vi "Get 430 Rate.vi"(5 "Field [T]":dbl, 7 "Override field?":bool, 8 "error in (no error)":errorcluster, 11 "VISA session":refnum<visa-resource-name>="GPIB0::22::INSTR") -> (0 "error out":errorcluster, 2 "Slew Rate [T/min]":dbl, 3 "VISA session out":refnum<visa-resource-name>="GPIB0::22::INSTR")   [LabVIEW 2021]
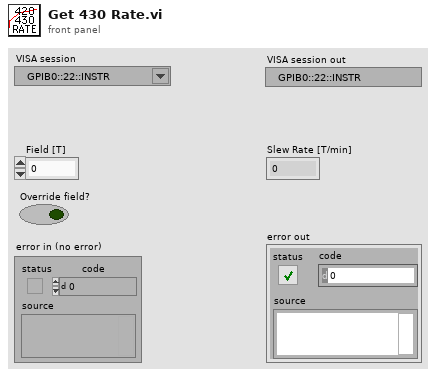
[diagram p1: front panel]
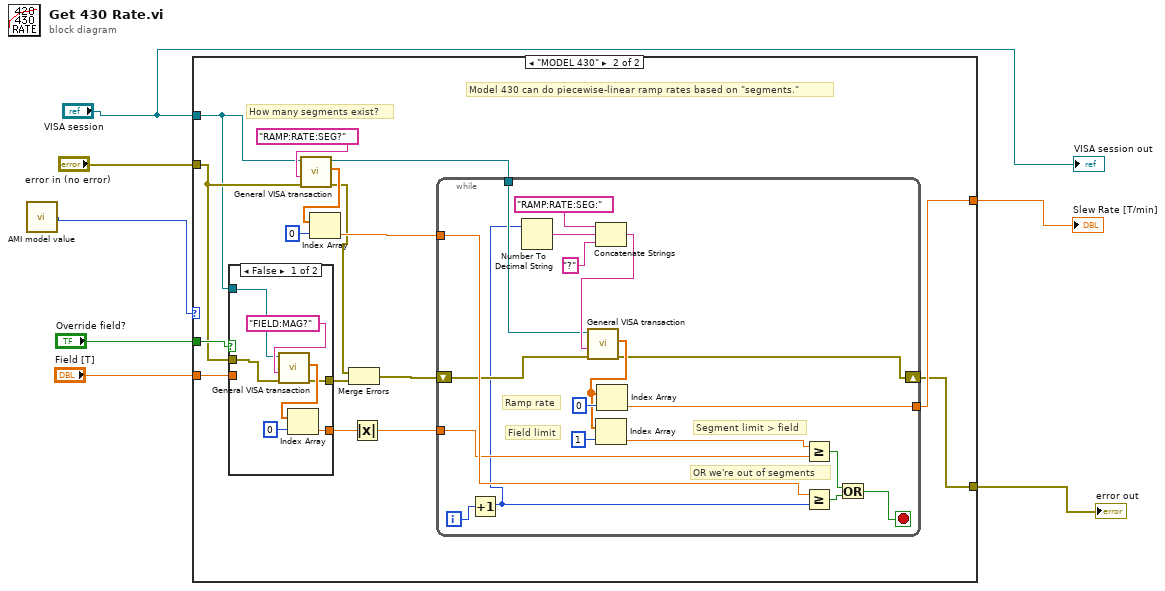
[diagram p0: block diagram]
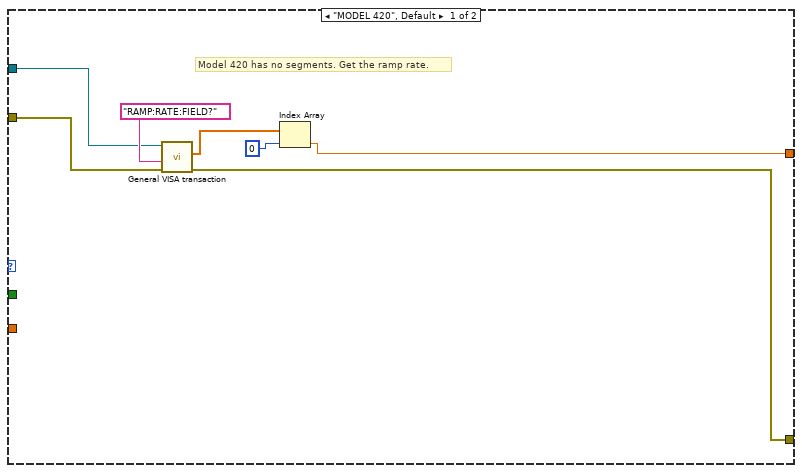
[diagram p2: hidden frame]
diagram:
  n1 = call "AMI model value.vi"() -> ("AMI Model 2"=w1:enum16{"MODEL 420", "MODEL 430"})  [unwired: 2 in]
  n2 = case shown="\"MODEL 430\"" w1 {
    tunnel: "VISA session" -> [w13 w20]
    tunnel: "error in (no error)" -> [w12 w25]
    tunnel: "Field [T]" -> [_ w29]
    tunnel: [w11 w15] -> w5
    tunnel: [w8 w16] -> w3
    tunnel: "Override field?" -> [_ w30]
    frame "MODEL 420", Default {
      # "Model 420 has no segments. Get the ramp rate."
      n3 = call "General VISA transaction.vi"("error in (no error)"=w12, "Command String"="RAMP:RATE:FIELD?", "VISA Session"=w13) -> ("error out"=w11:errorcluster, "Measurement"=w9:dbl[])  [unwired: 3 in, 4 out]
      n4 = Index Array(array=w9, index=0) -> (element=w8:dbl)
    }
    frame "MODEL 430" {
      # "How many segments exist?"
      # "Model 430 can do piecewise-linear ramp rates based on \"segments.\""
      n5 = case shown="False" w30 {
        tunnel: w29 -> [_ w58]
        tunnel: w25 -> [w55 w57]
        tunnel: [w52 w58] -> w18
        tunnel: [w51 w57] -> w23
        tunnel: w20 -> [w50 _]
        frame False {
          n6 = call "General VISA transaction.vi"("error in (no error)"=w55, "Command String"="FIELD:MAG?", "VISA Session"=w50) -> ("error out"=w51:errorcluster, "Measurement"=w53:dbl[])  [unwired: 3 in, 4 out]
          n7 = Index Array(array=w53, index=0) -> (element=w52:dbl)
        }
        frame True {
        }
      }
      n8 = call "General VISA transaction.vi"("error in (no error)"=w25, "Command String"="RAMP:RATE:SEG?", "VISA Session"=w20) -> ("error out"=w22:errorcluster, "Measurement"=w27:dbl[], "dup VISA Session"=w19:refnum<visa-resource-name>)  [unwired: 3 in, 3 out]
      n9 = Index Array(array=w27, index=0) -> (element=w24:dbl)
      n10 = Merge Errors(w22, w23) -> (w21:errorcluster)
      n11 = Absolute Value(x=w18) -> (abs(x)=w17:dbl)
      n12 = while {
        tunnel: w24 -> [w48]
        shift-right: [w33] -> w15
        shift-left: w21 -> [w39]
        tunnel: w19 -> [w40]
        tunnel: w17 -> [w35]
        tunnel: [w32] -> w16
        i -> [w49]
        stop <- w46 stop-if-true
        # "OR we're out of segments"
        # "Segment limit > field"
        # "Field limit"
        # "Ramp rate"
        n13 = Increment(x=w49) -> (x+1=w31:i32)
        n14 = Number To Decimal String(number=w31) -> (decimal integer string=w43:string)  [unwired: 1 in]
        n15 = Concatenate Strings("RAMP:RATE:SEG:" ("Command String"), w43, "?" ("Command String")) -> (w41:string)
        n16 = call "General VISA transaction.vi"("error in (no error)"=w39, "Command String"=w41, "VISA Session"=w40) -> ("error out"=w33:errorcluster, "Measurement"=w37:dbl[])  [unwired: 3 in, 4 out]
        n17 = Index Array(array=w37, index=1) -> (element=w36:dbl)
        n18 = Index Array(array=w37, index=0) -> (element=w32:dbl)
        n19 = Greater Or Equal?(x=w36, y=w35) -> (x >= y?=w34:bool)
        n20 = Greater Or Equal?(x=w48, y=w31) -> (x >= y?=w47:bool)
        n21 = Or(x=w34, y=w47) -> (x .or. y?=w46:bool)
      }
    }
  }
  "error out" <- w5
  "Slew Rate [T/min]" <- w3
  "VISA session out" <- "VISA session"
